vi "Open_Excel_Sequence.vi"(1 "Sheet name (optional)":string, 2 "Excel File Path":path) -> (0 "Sequence":cluster{string, string[], dbl[], dbl}[](array[cluster]))   [LabVIEW 2011]
doc: "This is an obselete VI designed to parse excel files and output a sequence array. The functionality remains available as an example implementation of an excel file parser."
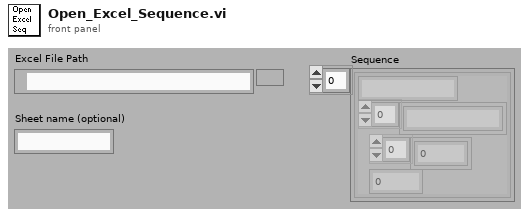
[diagram p1: front panel]
types:
  T1 = cluster{"Start Row":i32, "Start Column":i32, "End Row":i32, "End Column":i32}
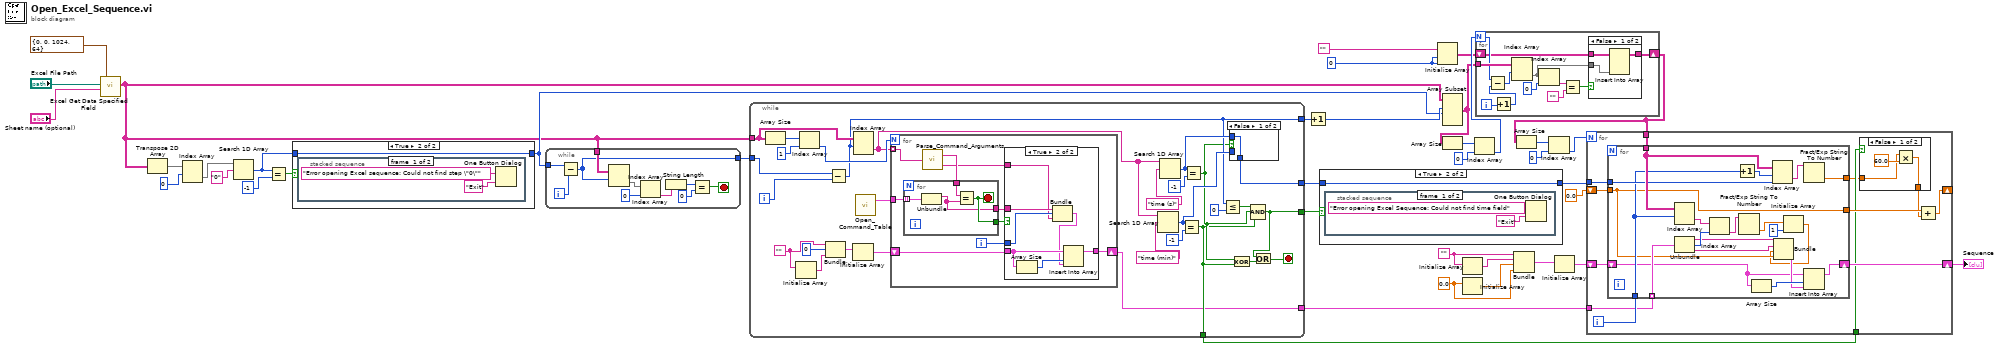
[diagram p0: block diagram]
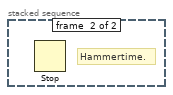
[diagram p6: hidden frame]
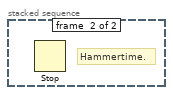
[diagram p9: hidden frame]
diagram:
  w3 = 0.0
  w4 = ""
  w18 = 0 ("dimension size")
  n1 = call "Excel Get Data Specified Field.vi"("SheetName"="Sheet name (optional)", "file path"="Excel File Path", "Start and End"=T1 {"Start Row"=0, "Start Column"=0, "End Row"=1024, "End Column"=64}) -> ("data"=w11:string[][])  [unwired: 1 in, 3 out]
  n2 = Transpose 2D Array(2D array=w11) -> (transposed array=w32:string[][])
  n3 = Index Array(array=w32, index (row)=0) -> (element=w33:string[])  [unwired: 1 in]
  n4 = Search 1D Array(1D array=w33, element="0") -> (index of element=w34:i32)  [unwired: 1 out]
  n5 = Equal?(x=w34, y=-1) -> (x = y?=w35:bool)
  n6 = case shown="True" w35 {
    tunnel: [w40 w41] -> w22
    tunnel: w34 -> [w40 w41]
    frame False {
    }
    frame True {
      n7 = stacked-sequence {
        frame #0 {
          n8 = One Button Dialog(message="Error opening Excel sequence: Could not find step \"0\"", button name ("OK")="Exit") -> ()  [unwired: 1 out]
        }
        frame #1 {
          # "Hammertime."
          n9 = Stop() -> ()  [unwired: 1 out]
        }
      }
    }
  }
  n10 = while {
    tunnel: w11 -> [w53]
    tunnel: w22 -> [w52]
    tunnel: [w44] -> w28
    i -> [w51]
    stop <- w47 stop-if-true
    n11 = Subtract(x=w52, y=w51) -> (x-y=w44:i32)
    n12 = Index Array(array=w53, index (row)=w44) -> (element=w46:string[])  [unwired: 1 in]
    n13 = Index Array(array=w46, index=0) -> (element=w48:string)
    n14 = String Length(string=w48) -> (length=w45:i32)
    n15 = Equal?(x=w45, y=0) -> (x = y?=w47:bool)
  }
  n16 = while {
    tunnel: w11 -> [w77]
    tunnel: [w66] -> w12
    tunnel: [w61] -> w30
    tunnel: [w73] -> w29
    tunnel: w28 -> [w68]
    tunnel: [w64] -> w23
    tunnel: [w59] -> w6
    i -> [w67]
    stop <- w65 stop-if-true
    w54 = ""
    n17 = Array Size(array=w77) -> (size(s)=w82:i32[])
    n18 = Initialize Array(w54) -> (w56:string[])  [unwired: 1 out]
    n19 = Index Array(array=w82, index=1) -> (element=w80:i32)
    n20 = Bundle(w54, 0, w56) -> (w57:cluster{string, i32, string[]})  [unwired: 1 out]
    n21 = Subtract(x=w68, y=w67) -> (x-y=w64:i32)
    n22 = Initialize Array(w57) -> (w58:cluster{string, i32, string[]}[])  [unwired: 1 out]
    n23 = Index Array(array=w77, index (row)=w64) -> (element=w74:string[])  [unwired: 1 in]
    n24 = call "Open_Command_Table.vi"() -> ("Commands"=w60:cluster{string, string[]}[])  [unwired: 2 out]
    n25 = for {
      N: w80 -> [_]
      tunnel: w60 -> [w93]
      tunnel: w74 -> [w87] mode=indexing
      shift-right: [w88] -> w59
      shift-left: w58 -> [w89]
      i -> [w90]
      n26 = call "Parse_Command_Arguments.vi"("Command String"=w87) -> ("Command"=w86:string, "Argument List"=w85:string[])
      n27 = for {
        tunnel: w93 -> [w105] mode=indexing
        tunnel: w86 -> [w104]
        tunnel: [w103] -> w92
        tunnel: [w102] -> w91
        stop <- w103 stop-if-true
        n28 = Unbundle(w105) -> (w102:string)  [unwired: 1 out]
        n29 = Equal?(x=w104, y=w102) -> (x = y?=w103:bool)
      }
      n30 = case shown="True" w92 {
        tunnel: w91 -> [_ w101]
        tunnel: w90 -> [_ w100]
        tunnel: w89 -> [w94 w98]
        tunnel: [w94 w96] -> w88
        tunnel: w85 -> [_ w95]
        frame False {
        }
        frame True {
          n31 = Array Size(array=w98) -> (size(s)=w99:i32)
          n32 = Bundle(w101, w100, "Argument List"=w95) -> (w97:cluster{string, i32, "Argument List":string[]})  [unwired: 1 out]
          n33 = Insert Into Array(array=w98, index=w99, new element=w97) -> (w96:cluster{string, i32, string[]}[])
        }
      }
    }
    n34 = Search 1D Array(1D array=w74, element="time (min)") -> (index of element=w71:i32)  [unwired: 1 out]
    n35 = Search 1D Array(1D array=w74, element="time (s)") -> (index of element=w72:i32)  [unwired: 1 out]
    n36 = Equal?(x=w71, y=-1) -> (x = y?=w61:bool)
    n37 = Equal?(x=w72, y=-1) -> (x = y?=w62:bool)
    n38 = Less Or Equal?(x=w64, y=0) -> (x <= y?=w69:bool)
    n39 = case shown="False" w62 {
      tunnel: [w83 w84] -> w73
      tunnel: w72 -> [w83 _]
      tunnel: w71 -> [_ w84]
      frame False {
      }
      frame True {
      }
    }
    n40 = Exclusive Or(1:w61, 2:w62) -> (0:w63:bool)
    n41 = Compound Arithmetic op=AND(w69, w62, w61) -> (w66:bool)
    n42 = Or(x=w66, y=w63) -> (x .or. y?=w65:bool)
  }
  n43 = Increment(x=w23) -> (x+1=w24:i32)
  n44 = case shown="True" w12 {
    tunnel: [w106 w107] -> w27
    tunnel: w29 -> [w106 w107]
    frame False {
    }
    frame True {
      n45 = stacked-sequence {
        frame #0 {
          n46 = One Button Dialog(message="Error opening Excel Sequence: Could not find time field", button name ("OK")="Exit") -> ()  [unwired: 1 out]
        }
        frame #1 {
          # "Hammertime."
          n47 = Stop() -> ()  [unwired: 1 out]
        }
      }
    }
  }
  n48 = Initialize Array("", w18, w18) -> (w17:string[][])
  n49 = Array Subset(array=w11, index (row)=w24, length (row)=w22) -> (w20:string[][])  [unwired: 2 in]
  n50 = Array Size(array=w20) -> (size(s)=w26:i32[])
  n51 = Initialize Array(w4) -> (w5:string[])  [unwired: 1 out]
  n52 = Initialize Array(w3) -> (w2:dbl[])  [unwired: 1 out]
  n53 = Index Array(array=w26, index=0) -> (element=w21:i32)
  n54 = for {
    N: w21 -> [w120]
    tunnel: w20 -> [w121]
    shift-right: [w112] -> w14
    shift-left: w17 -> [w113]
    i -> [w111]
    n55 = Increment(x=w111) -> (x+1=w110:i32)
    n56 = Subtract(x=w120, y=w110) -> (x-y=w119:i32)
    n57 = Index Array(array=w121, index (row)=w119) -> (element=w114:string[])  [unwired: 1 in]
    n58 = Index Array(array=w114, index=0) -> (element=w117:string)
    n59 = Equal?(x=w117, y="") -> (x = y?=w115:bool)
    n60 = case shown="False" w115 {
      tunnel: w114 -> [w122 _]
      tunnel: w113 -> [w124 w125]
      tunnel: [w123 w125] -> w112
      frame False {
        n61 = Insert Into Array(array=w124, new element=w122) -> (w123:string[][])  [unwired: 2 in]
      }
      frame True {
      }
    }
  }
  n62 = Bundle(w4, w5, w2, w3) -> (w8:cluster{string, string[], dbl[], dbl})  [unwired: 1 out]
  n63 = Array Size(array=w14) -> (size(s)=w16:i32[])
  n64 = Index Array(array=w16, index=0) -> (element=w13:i32)
  n65 = Initialize Array(w8) -> (w7:cluster{string, string[], dbl[], dbl}[])  [unwired: 1 out]
  n66 = for {
    N: w13 -> [_]
    shift-right: [w137] -> w1
    shift-left: w7 -> [w136]
    tunnel: w14 -> [w135]
    tunnel: w27 -> [w133]
    shift-right: [w130] -> _
    shift-left: 0.0 -> [w132]
    tunnel: w30 -> [w129]
    tunnel: w6 -> [w126]
    i -> [w134]
    n67 = for {
      shift-right: [w145] -> w137
      shift-left: w136 -> [w146]
      tunnel: w135 -> [w161]
      tunnel: w134 -> [w156]
      tunnel: w133 -> [w160]
      tunnel: w132 -> [w151]
      tunnel: [w151] -> w131
      tunnel: [w158] -> w128
      tunnel: w126 -> [w155] mode=indexing
      n68 = Index Array(array=w161, index (row)=w156) -> (element=w153:string[])  [unwired: 1 in]
      n69 = Unbundle(w155) -> (w149:string, w154:i32, w148:string[])
      n70 = Index Array(array=w153, index=w154) -> (element=w150:string)
      n71 = Increment(x=w156) -> (x+1=w157:i32)
      n72 = Fract/Exp String To Number(string=w150) -> (number=w143:dbl)  [unwired: 4 out]
      n73 = Array Size(array=w146) -> (size(s)=w152:i32)
      n74 = Index Array(array=w161, index (row)=w157, index (col)=w160) -> (element=w159:string)
      n75 = Initialize Array(w143, 1 ("dimension size")) -> (w142:dbl[])
      n76 = Bundle(w149, w148, w142, w151) -> (w147:cluster{string, string[], dbl[], dbl})  [unwired: 1 out]
      n77 = Fract/Exp String To Number(string=w159) -> (number=w158:dbl)  [unwired: 4 out]
      n78 = Insert Into Array(array=w146, index=w152, new element=w147) -> (w145:cluster{string, string[], dbl[], dbl}[])
    }
    n79 = case shown="False" w129 {
      tunnel: w128 -> [w139 w141]
      tunnel: [w138 w141] -> w127
      frame False {
        n80 = Multiply(x=w139, y=60.0) -> (x*y=w138:dbl)
      }
      frame True {
      }
    }
    n81 = Add(x=w131, y=w127) -> (x+y=w130:dbl)
  }
  "Sequence" <- w1
